vi "Blob FromImages.vi"(0 "Blob":refnum<class "Blob.lvclass">, 1 "ScaleFactor":dbl=1.0, 3 "Mean":dbl[](array[numeric]), 5 "images":T1[](array[typedef]), 7 "Size":T3, 11 "error in":errorcluster, 12 "DDepth":T2=enum."CV_32F", 13 "SwapRB":bool, 14 "Crop":bool) -> (4 "Blob out":refnum<class "Blob.lvclass">, 15 "error out":errorcluster)   [LabVIEW 2020, in "OpenLvVision_OpenCv.lvlib" / "Blob.lvclass"]
doc: "Creates 4-dimensional blob from series of images. Optionally resizes and crops images from center, subtract mean values, scales values by scalefactor, swap Blue and Red channels."
uses:
  Blob.lvclass
  TypeDef/Point/2D_PointI32.ctl
  C:/Users/lukas/Downloads/OpenLvVision_OpenCv/SourceCode/LabView/OpenLvVision_OpenCv/_LvHelpers/EdvrObject/EdvrObject.lvclass
  TypeDef/NchwType.ctl
  <vilib>/vision/Image Controls.llb/IMAQ Image.ctl
  _LvHelpers/EdvrObject/EdvrObject.lvclass/EdvrObject.ctl
  _LvHelpers/MatHandling/RegisterMat/RegisterMat_Image.vi
  _LvHelpers/MatHandling/UnregisterMat/UnregisterMat_Image.vi
  OpenLvVision_OpenCv.lvlib
  _LvHelpers/EdvrObject/EdvrObject.lvclass
  Dlls/OlvOpenCvWrapper.dll
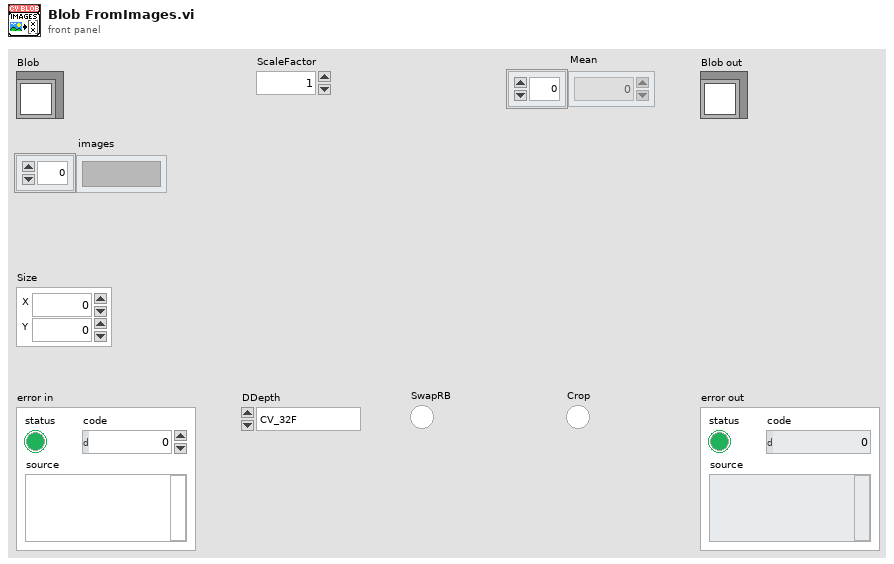
[diagram p1: front panel]
types:
  T1 = typedef "IMAQ Image.ctl" = refnum<image>
  T2 = typedef "OpenLvVision_OpenCv.lvlib/NchwType.ctl" = enum16{"CV_U8", "CV_8S", "CV_16U", "CV_16S", "CV_32S", "CV_32F", "CV_64F", "CV_16F"}
  T3 = typedef "OpenLvVision_OpenCv.lvlib/2D_PointI32.ctl" = cluster{"X":i32, "Y":i32}
  T4 = typedef "OLV OpenLvVision_Image.lvlib/OLV Management.lvlib/OLV Image.ctl" = refnum<image>
  T5 = typedef "OpenLvVision_OpenCv.lvlib/MatInfo.ctl" = cluster{"Datatype":T6, "Height":i32, "Width":i32, "Channels":i32, "LineWidth":i32, "Null":u8}
  T6 = typedef "OpenLvVision_OpenCv.lvlib/LvDatatype.ctl" = enum32{"Undefined", "U8", "I8", "U16", "I16", "U32_Color", "I32", "U64_Color", "I64", "SGL", "DBL", "Complex SGL", "Complex DBL", "Array 1D U8", "Array 1D I8", "Array 1D U16", "Array 1D I16", "Array 1D U32_Color", "Array 1D I32", "Array 1D U64_Color", "Array 1D I64", "Array 1D SGL", "Array 1D DBL", "Array 1D Complex SGL", "Array 1D Complex DBL", "Array 2D U8", "Array 2D I8", "Array 2D U16", "Array 2D I16", "Array 2D U32", "Array 2D U32_Color", "Array 2D I32", "Array 2D U64", "Array 2D U64_Color", "Array 2D I64", "Array 2D SGL", "Array 2D DBL", "Array 2D Complex SGL", "Array 2D Complex DBL", "Image Mono U8", "Image Mono U16", "Image Mono I16", "Image Mono SGL", "Image Color U32", "Image Color U64", "ImageComplex Sgl", "Array1d_2dPointI32", "Array1d_2dPointSGL", "Array1d_2dPointDBL", "Array1d_3dPointI32", "Array1d_3dPointSGL", "Array1d_3dPointDBL", "Array1d_4dPointI32", "Array1d_4dPointSGL", "Array1d_4dPointDBL", "ArrayNchwU8", "ArrayNchwI8", "ArrayNchwU16", "ArrayNchwI16", "ArrayNchwU32_Color", "ArrayNchwI32", "ArrayNchwU64_Color", "ArrayNchwSgl", "ArrayNchwDbl", "ArrayNchwComplexSgl", "ArrayNchwComplexDbl"}
  T7 = typedef "OpenLvVision_OpenCv.lvlib/EdvrObject.lvclass/Edvr.ctl" = refnum<data-value>
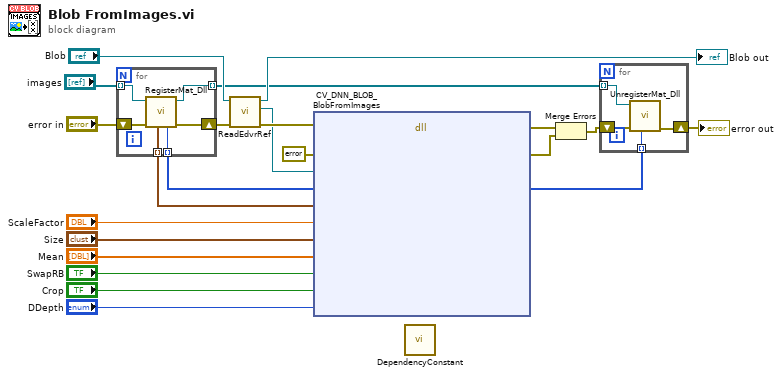
[diagram p0: block diagram]
diagram:
  n1 = for {
    tunnel: [w28] -> w17 mode=indexing
    shift-right: [w26] -> w10
    shift-left: "error in" -> [w27]
    tunnel: "images" -> [w25] mode=indexing
    tunnel: [w24] -> w6 mode=indexing
    tunnel: [w23] -> w8 mode=indexing
    n2 = call-poly "RegisterMat_Dll.vi"("error in"=w27, "Image Reference In"=w25) -> ("error out"=w26:errorcluster, "Image Reference Out"=w24:T4, "AdressOrData"=w23:u64, "Mat"=w28:T5)  [unwired: 6 in]
  }
  n3 = call "ReadEdvrRef.vi"("error in (no error)"=w10, "EdvrObject in"="Blob") -> ("error out"=w16:errorcluster, "Edvr"=w15:T7, "EdvrObject out"=→"Blob out":refnum<class "Blob.lvclass">)  [unwired: 7 in]
  n4 = dll-call lib="C:/Users/lukas/Downloads/OpenLvVision_OpenCv/SourceCode/LabView/OpenLvVision_OpenCv/Dlls/OlvOpenCvWrapper.dll" fn="CV_DNN_BLOB_BlobFromImages"(error in=w16, "Error"=errorcluster {"status"=FALSE, "code"=0, "source"=""} ("error constant"), "edvrRef"=w15, "AdressImages"=w8, "MatInfoImages"=w17, "scalefactor"="ScaleFactor", "size"="Size", "meanHandle"="Mean", "swapRB"="SwapRB", "crop"="Crop", "ddepth"="DDepth") -> (error out=w21:errorcluster, "Error"=w20:errorcluster, "AdressImages"=w4:u64[])  [unwired: 11 in, 1 out]
  n5 = call "DependencyConstant.vi"() -> ()  [unwired: 12 in]
  n6 = Merge Errors(w21, w20) -> (w7:errorcluster)
  n7 = for {
    shift-right: [w30] -> w5
    shift-left: w7 -> [w31]
    tunnel: w6 -> [w32] mode=indexing
    tunnel: w4 -> [w29] mode=indexing
    n8 = call-poly "UnregisterMat_Dll.vi"("AdressOrData"=w29, "error in"=w31, "Image Reference In"=w32) -> ("error out"=w30:errorcluster)  [unwired: 7 in, 1 out]
  }
  "error out" <- w5
